vi "DriveAutonomous.vi"(6 "GyroData":T1, 9 "Rotation":dbl, 10 "LY_Axis":dbl, 11 "LX_Axis":dbl) -> (0 "error out":errorcluster, 1 "Y_AxisCmd":dbl, 2 "X_AxisCmd":dbl, 3 "Motor Values":dbl[](array[numeric]), 5 "RotationCmd":dbl)   [LabVIEW 2017]
uses:
  Support Code/Gyro/Gyro_TypeDef.ctl
  <vilib>/Rock Robotics/WPI/Utilities/WPI_GetSetVariantRefNum.vi
  <vilib>/Rock Robotics/WPI/RobotDrive/WPI_RobotDriveMecanumDrive_Cartesian.vi
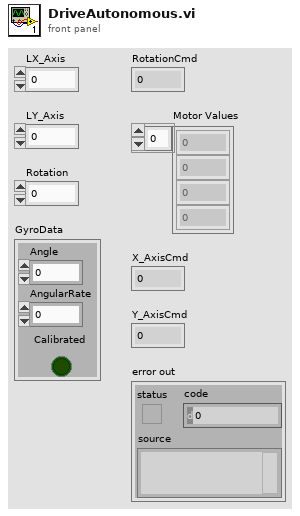
[diagram p1: front panel]
types:
  T1 = typedef "Gyro_TypeDef.ctl" = cluster{"Angle":dbl, "AngularRate":dbl, "Calibrated":bool}
  T2 = typedef "WPI_RobotDriveDevRef.ctl" = cluster{"DevStatus":errorcluster, "Motors[]":T3[], "Square Inputs":bool, "Max Output":dbl}
  T3 = typedef "WPI_MotorControlDeviceRef.ctl" = cluster{"DeviceStatus":errorcluster, "Type":T4, "PWM":cluster{"PWM Channel":T5, "DeadBand":T6}, "CAN":cluster{"Device Number":u8, "SetOutput VI Ref":variant, "GetOutput VI Ref":variant, "Enable VI Ref":variant, "Disable VI Ref":variant, "Data":variant}, "Invert":bool, "DIO PWM":cluster{"PWM \"Enable\" Channel":T5, "DIOChannel":T7, "PWM Rate":dbl}}
  T4 = typedef "WPI_MotorControlType.ctl" = enum16{"PWM", "CAN", "DIO PWM"}
  T5 = typedef "FPGA_DIOPWMChannel.ctl" = enum8{"PWM 0", "PWM 1", "PWM 2", "PWM 3", "PWM 4", "PWM 5", "PWM 6", "PWM 7", "PWM 8", "PWM 9", "PWM MXP 0", "PWM MXP 1", "PWM MXP 2", "PWM MXP 3", "PWM MXP 4", "PWM MXP 5", "PWM MXP 6", "PWM MXP 7", "PWM MXP 8", "PWM MXP 9", "Invalid"}
  T6 = typedef "WPI_PWMDeadband.ctl" = cluster{"Name":string, "maxPositivePwm":i32, "minPositivePwm":i32, "centerPwm":i32, "maxNegativePwm":i32, "minNegativePwm":i32, "angularRange":u16}
  T7 = typedef "FPGA_DIOChannel.ctl" = enum8{"DIO 0", "DIO 1", "DIO 2", "DIO 3", "DIO 4", "DIO 5", "DIO 6", "DIO 7", "DIO 8", "DIO 9", "DIO MXP 0", "DIO MXP 1", "DIO MXP 2", "DIO MXP 3", "DIO MXP 4", "DIO MXP 5", "DIO MXP 6", "DIO MXP 7", "DIO MXP 8", "DIO MXP 9", "DIO MXP 10", "DIO MXP 11", "DIO MXP 12", "DIO MXP 13", "DIO MXP 14", "DIO MXP 15", "SPI Port CS1", "SPI Port CS2", "SPI Port CS3", "SPI Port MISO", "SPI Port MOSI", "Invalid"}
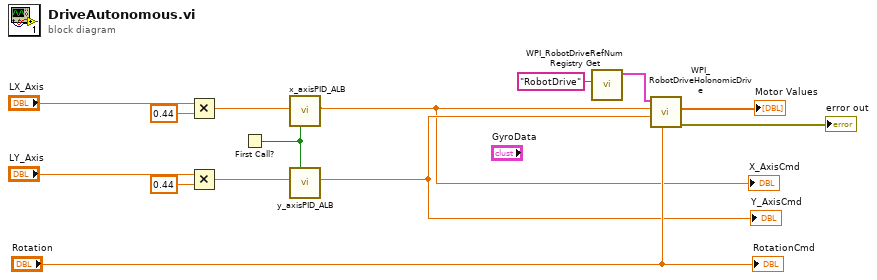
[diagram p0: block diagram]
diagram:
  n1 = Multiply(x="LX_Axis", y=0.44) -> (x*y=w7:dbl)
  n2 = Multiply(x="LY_Axis", y=0.44) -> (x*y=w9:dbl)
  n3 = First Call?() -> (First Call?: T/F=w11:bool)
  n4 = call "x_axisPID_ALB.vi"("First Call?: T/F"=w11, "x axis"=w7) -> ("x axis out"=w8:dbl)  [unwired: 9 in]
  "X_AxisCmd" <- w8
  n5 = call "y_axisPID_ALB.vi"("First Call?: T/F"=w11, "y axis"=w9) -> ("y axis out"=w10:dbl)  [unwired: 9 in]
  "Y_AxisCmd" <- w10
  n6 = call <vilib>:"WPI_RobotDriveRefNum Registry Get.vi"("refnum name"="RobotDrive") -> ("RobotDriveDevRef"=w5:T2)  [unwired: 9 in, 1 out]
  n7 = call-poly <vilib>:"WPI_RobotDriveHolonomicDrive.vi"("Rotation"="Rotation", "Y"=w10, "X"=w8, "RobotDriveDevRef"=w5) -> ("error out"=→"error out":errorcluster, "Motor Values"=→"Motor Values":dbl[])  [unwired: 5 in, 1 out]
  "RotationCmd" <- "Rotation"
